vi "Configure Export Signal.vi"(8 "error in":errorcluster, 11 "FGen PXI Base CFG in":refnum<class "FGen PXI Base CFG.lvclass">) -> (0 "error out":errorcluster, 3 "FGen PXI Base CFG out":refnum<class "FGen PXI Base CFG.lvclass">)   [LabVIEW 2023, in "FGen PXI Base CFG.lvlib" / "FGen PXI Base CFG.lvclass"]
uses:
  FGen PXI Base CFG.lvclass
  <instrlib>/niFgen/niFgen.llb/niFgen_ctl Exported Signal Name Values (Ring).ctl
  <instrlib>/niFgen/niFgen.llb/niFgen_ctl Exported Signal Identifiers (Ring).ctl
  <instrlib>/niFgen/niFgen.llb/niFgen_ctl Exported Signal Desination Values (ComboBox).ctl
  Configuration/Configuration JSON/Configuration JSON Base/CFG JSON.lvclass/CFG JSON.ctl
  FGen PXI Base CFG.lvclass/FGen PXI Base CFG.ctl
  6833aab5-89e2-4c30-8132-47a66f565ddb.vi
  <vilib>/JDP Science/JSONtext/Find Item.vi
  <vilib>/JDP Science/JSONtext/Next JSON Value.vi
  <vilib>/JDP Science/JSONtext/String Subset.vi
  <vilib>/JDP Science/JSONtext/Parsing/Advance past next JSON Value (inlined COPY).vi
  <vilib>/JDP Science/JSONtext/Parsing/Advance past whitespace.vi
  <vilib>/JDP Science/JSONtext/Parsing/Advance past String.vi
  <vilib>/JDP Science/JSONtext/Parsing/Advance past Number.vi
  <vilib>/JDP Science/JSONtext/Parsing/Advance past Line Ending.vi
  <vilib>/JDP Science/JSONtext/Parsing/Parse Full Path or Item Name.vi
  <vilib>/JDP Science/JSONtext/Parsing/Advance past Array.vi
  <vilib>/JDP Science/JSONtext/Parsing/Advance past Object.vi
  <vilib>/JDP Science/JSONtext/support/Error Cluster From Code.vi
  <vilib>/JDP Science/JSONtext/Offset/Find Item Locations by Path.vi
  <vilib>/JDP Science/JSONtext/JSON text to Variant.vi
  <vilib>/Utility/error.llb/Error Cluster From Error Code.vi
  <vilib>/JDP Science/JSONtext/LVClass Serializer/JSONtext LVClass Serializer.lvclass
  <vilib>/ErrorRing/Error Ring.xnode
  Configuration/Configuration JSON/Configuration JSON Base/CFG JSON.lvclass
panel:
  out "Output Terminal":T1="PFI0" caption="output terminal (do not export)"
  out "Signal Identifier":T2 caption="Signal Identifier (None)"
  out "Signal":T3=1002 caption="Signal (Marker Event)" items=["Sample Clock"=101, "Sample Clock Timebase"=1006, "Reference Clock"=102, "Onboard Reference Clock"=1019, "Start Trigger"=1004, "Script Trigger"=103, "Marker Event"=1001, "Data Marker Event"=108, "Ready For Start Event"=105, "Started Event"=106, "Done Event"=107, "Synchronization Pulse"=1007, "Sync Out"=1002]
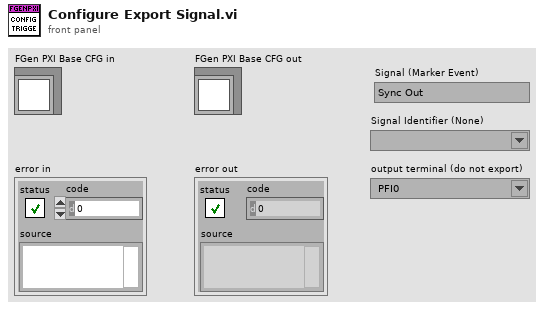
[diagram p1: front panel]
types:
  T1 = typedef "niFgen_ctl Exported Signal Desination Values (ComboBox).ctl" = string
  T2 = typedef "niFgen_ctl Exported Signal Identifiers (Ring).ctl" = string
  T3 = typedef "niFgen_ctl Exported Signal Name Values (Ring).ctl" = u16
  T4 = cluster{"Enabled":bool, "Output Terminal":string, "Signal Identifier":string, "Signal":string}
  T5 = typedef "LVComboBoxStrsAndValuesArrayTypeDef.ctl" = cluster{"String":string, "Value":string}[]
  T6 = typedef "LVStringsAndValuesArrayTypeDef_U16.ctl" = cluster{"String":string, "Value":u16}[]
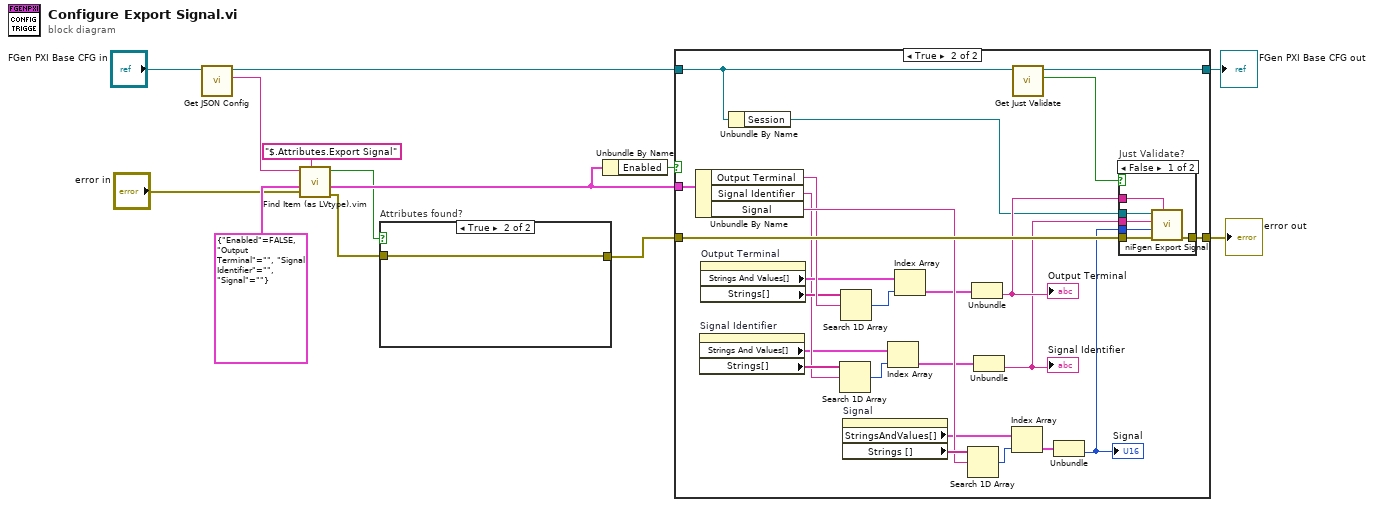
[diagram p0: block diagram]
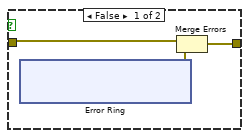
[diagram p2: hidden frame]
diagram:
  n1 = call "Get JSON Config.vi"("CFG Base in"="FGen PXI Base CFG in") -> ("<JSON>Config>"=w9:string, "CFG Base out"=w2:refnum<class "FGen PXI Base CFG.lvclass">)  [unwired: 9 in]
  n2 = call "Find Item (as LVtype).vim"("$Path or Item Name"="$.Attributes.Export Signal", "error in (no error)"="error in", "Data Type and Default Value"=T4 {"Enabled"=FALSE, "Output Terminal"="", "Signal Identifier"="", "Signal"=""}, "JSON"=w9) -> ("error out"=w6:errorcluster, "Data"=w7:T4, "Found"=w5:bool)  [unwired: 4 in, 1 out]
  n3 = case "Attributes found?" shown="True" w5 {
    tunnel: [w16 w22] -> w4
    tunnel: w6 -> [w15 w22]
    frame False {
      n4 = xnode "Error Ring"() -> ("error out"=w14:errorcluster)
      n5 = Merge Errors(w15, w14) -> (w16:errorcluster)
    }
    frame True {
    }
  }
  n6 = Unbundle By Name(w7) -> ("Enabled"=w8:bool)
  n7 = case shown="True" w8 {
    tunnel: [w24 w47] -> w13
    tunnel: w4 -> [w24 w48]
    tunnel: w7 -> [_ w49]
    tunnel: w2 -> [w23 w27]
    tunnel: [w23 w25] -> w3
    frame False {
    }
    frame True {
      n8 = Unbundle By Name(w49) -> ("Output Terminal"=w40:string, "Signal Identifier"=w34:string, "Signal"=w45:string)
      n9 = property on="Signal Identifier" class="CmbBox (strict)"() -> ("Strings And Values[]"=w33:T5, "Strings[]"=w35:string[])  [unwired: 2 in, 2 out]
      n10 = property on="Output Terminal" class="CmbBox (strict)"() -> ("Strings And Values[]"=w38:T5, "Strings[]"=w39:string[])  [unwired: 2 in, 2 out]
      n11 = Unbundle By Name(w27) -> ("Session"=w28:refnum<k15>)
      n12 = Search 1D Array(1D array=w35, element=w34) -> (index of element=w32:i32)  [unwired: 1 in]
      n13 = Search 1D Array(1D array=w39, element=w40) -> (index of element=w37:i32)  [unwired: 1 in]
      n14 = property on="Signal" class="Ring (strict)"() -> ("StringsAndValues[]"=w44:T6, "Strings []"=w46:string[])  [unwired: 2 in, 2 out]
      n15 = Index Array(array=w33, index=w32) -> (element=w31:cluster{"String":string, "Value":string})
      n16 = Index Array(array=w38, index=w37) -> (element=w36:cluster{"String":string, "Value":string})
      n17 = Search 1D Array(1D array=w46, element=w45) -> (index of element=w43:i32)  [unwired: 1 in]
      n18 = Unbundle(w36) -> ("Value"=w30:string)  [unwired: 1 out]
      "Output Terminal" <- w30
      n19 = Unbundle(w31) -> ("Value"=w29:string)  [unwired: 1 out]
      "Signal Identifier" <- w29
      n20 = Index Array(array=w44, index=w43) -> (element=w42:cluster{"String":string, "Value":u16})
      n21 = call "Get Just Validate.vi"("CFG JSON Base in"=w27) -> ("Just Validate"=w26:bool, "CFG JSON Base out"=w25:refnum<class "FGen PXI Base CFG.lvclass">)  [unwired: 9 in]
      n22 = Unbundle(w42) -> ("Value"=w41:u16)  [unwired: 1 out]
      "Signal" <- w41
      n23 = case "Just Validate?" shown="False" w26 {
        tunnel: w48 -> [w55 w56]
        tunnel: [w54 w56] -> w47
        tunnel: w41 -> [w53 _]
        tunnel: w30 -> [w52 _]
        tunnel: w29 -> [w51 _]
        tunnel: w28 -> [w50 _]
        frame False {
          n24 = call <instrlib>:"niFgen Export Signal.vi"("Output Terminal (do not export)"=w52, "error in (no error)"=w55, "Signal"=w53, "Signal Identifier (None)"=w51, "Instrument Handle"=w50) -> ("error out"=w54:errorcluster)  [unwired: 5 in, 1 out]
        }
        frame True {
        }
      }
    }
  }
  "error out" <- w13
  "FGen PXI Base CFG out" <- w3
